vi "Append Report Text (str).vi"(0 "report in":refnum<class "NI_HTML.lvclass">, 1 "MS Office parameters":T1, 2 "format string (%.3f)":string="%.3f", 7 "text":string, 9 "append on new line? (F)":bool, 11 "error in (no error)":errorcluster) -> (4 "report out":refnum<class "NI_HTML.lvclass">, 8 "start out (Word)":i32, 10 "end out (Word)":i32, 15 "error out":errorcluster)   [LabVIEW 2017, in "NI_HTML.lvclass"]
doc: "Appends text to the selected report."
uses:
  <vilib>/Utility/NIReport.llb/HTML/NI_HTML.lvclass
  <vilib>/Utility/NIReport.llb/HTML/NI_HTML.lvclass/NI_HTML.ctl
  <vilib>/Utility/NIReport.llb/NI_ReportGenerationCore.lvlib
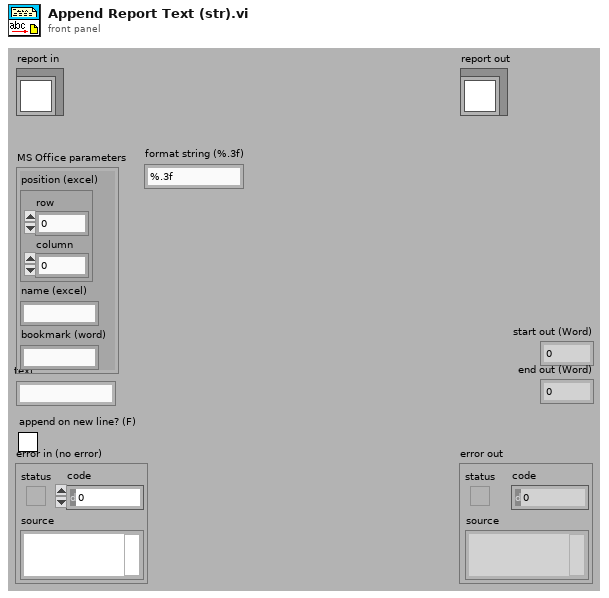
[diagram p1: front panel]
types:
  T1 = cluster{"position (excel)":cluster{"row":i32, "column":i32}, "name (excel)":string, "bookmark (word)":string}
  T2 = typedef "NI_ReportGenerationCore.lvlib/HTML Report Data.ctl" = cluster{"Body Text":string, "Font Tag":string, "Title Text":string, "Header Text":string, "Footer Text":string, "Image List":path[]}
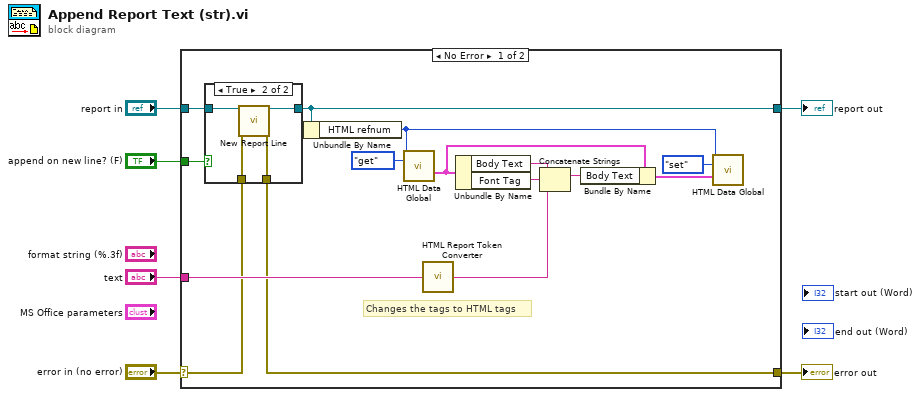
[diagram p0: block diagram]
diagram:
  n1 = case shown="No Error" "error in (no error)" {
    selector: "error in (no error)" -> [w14 w29]
    tunnel: [w13 w29] -> w5
    tunnel: [w11 w28] -> w3
    tunnel: "report in" -> [w16 w28]
    tunnel: "text" -> [w17 _]
    tunnel: "append on new line? (F)" -> [w15 _]
    frame No Error {
      # "Changes the tags to HTML tags"
      n2 = case shown="True" w15 {
        tunnel: w16 -> [w23 w27]
        tunnel: [w23 w26] -> w11
        tunnel: w14 -> [w22 w25]
        tunnel: [w22 w24] -> w13
        frame False {
        }
        frame True {
          n3 = call-dynamic "New Report Line.vi"("report in"=w27, "error in (no error)"=w25) -> ("report out"=w26:refnum<class "NI_HTML.lvclass">, "error out"=w24:errorcluster)  [unwired: 1 in, 11 out]
        }
      }
      n4 = Unbundle By Name(w11) -> ("HTML refnum"=w7:u32)
      n5 = call <vilib>:"HTML Data Global.vi"("HTML refnum"=w7, "menu"=enum16{"init", "get", "set", "delete"}."get") -> ("HTML report data out"=w8:T2)  [unwired: 1 in, 12 out]
      n6 = call <vilib>:"HTML Report Token Converter.vi"("String In"=w17) -> ("String Out"=w18:string)
      n7 = Unbundle By Name(w8) -> ("Body Text"=w21:string, "Font Tag"=w20:string)
      n8 = Concatenate Strings(w21, w20, w18) -> (w19:string)
      n9 = Bundle By Name(cluster=w8, "Body Text"=w19) -> (w9:T2)
      n10 = call <vilib>:"HTML Data Global.vi"("HTML refnum"=w7, "menu"=enum16{"init", "get", "set", "delete"}."set", "HTML report data in"=w9) -> ()  [unwired: 13 out]
    }
    frame Error {
    }
  }
  "error out" <- w5
  "report out" <- w3
